vi "test_harness_Sat_op_fxp_16_5.vi"() -> ()   [LabVIEW 2017, in "Sat_Hyst_TestCase.lvclass"]
uses:
  Sat_Hyst_TestCase.lvclass
  C:/Program Files (x86)/National Instruments/LabVIEW 2017/vi.lib/addons/_JKI Toolkits/VI Tester/TestCase.llb/TestCase.lvclass
  <vilib>/rvi/DesktopExecutionNode/Execution/niFpgaDEN_Execute.vi
  <vilib>/rvi/DesktopExecutionNode/DesktopExecutionNode.xnode
  <userlib>/_VITAC/VITAC.lvlib
panel:
  in  "error in (no error)":errorcluster
  out "error out":errorcluster
  out "TestCase out":refnum<class "Sat_Hyst_TestCase.lvclass">
  in  "TestCase in":refnum<class "Sat_Hyst_TestCase.lvclass">
  out "H_of_uk":fxp<+/-,32,10>[](array[numeric])
  out "sat(U) (expected, ML)":dbl[](array[numeric])
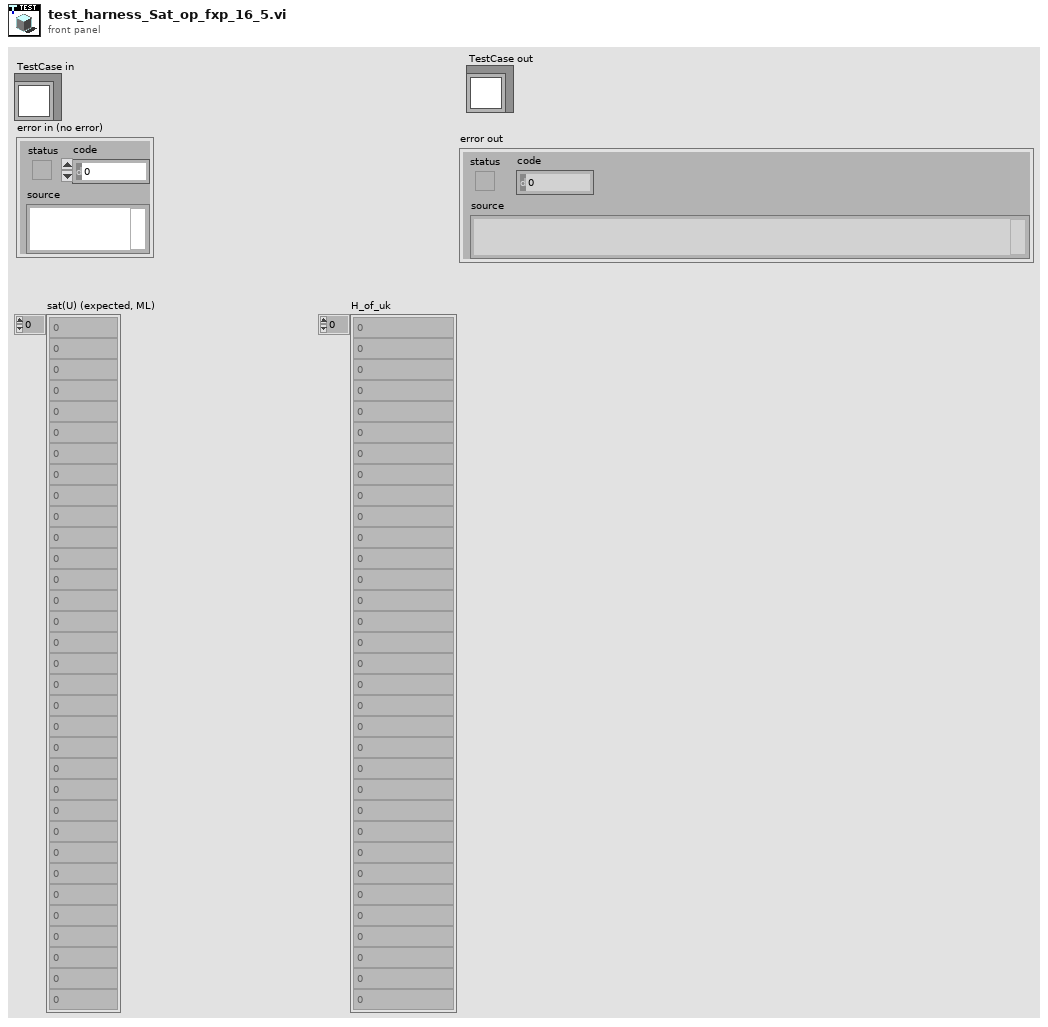
[diagram p1: front panel]
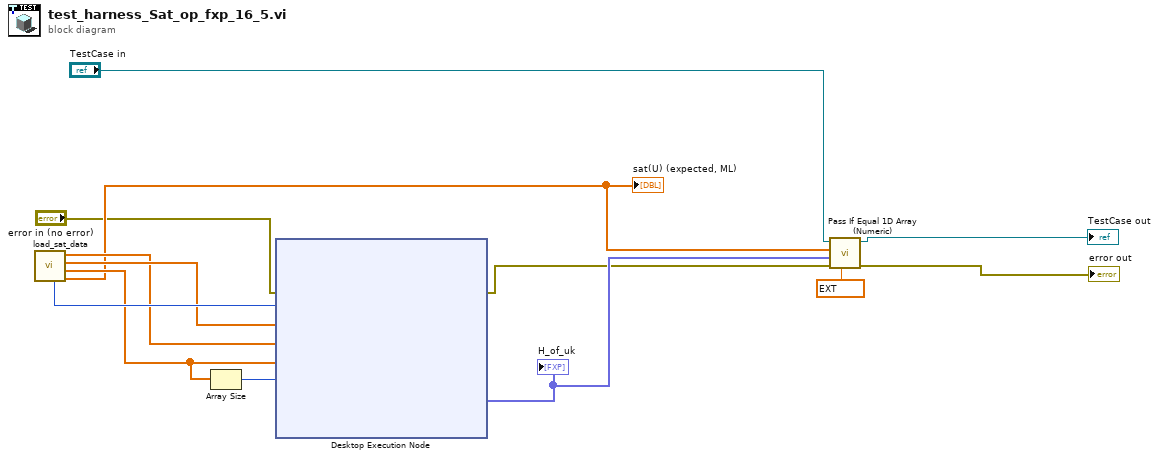
[diagram p0: block diagram]
diagram:
  n1 = call "load_sat_data.vi"() -> ("sat(U_nom)"=w6:dbl[], "U_nom"=w9:dbl[], "wsp"=w12:dbl[], "dps"=w11:dbl[], "N_hyst"=w13:i32)  [unwired: 7 in]
  "sat(U) (expected, ML)" <- w6
  n2 = Array Size(array=w9) -> (size(s)=w10:i32)
  n3 = xnode "Desktop Execution Node"("Error In"="error in (no error)", "N_sat"=w13, "satw_s"=w12, "d_s"=w11, "uk"=w9, "numIter"=w10) -> ("Error Out"=w3:errorcluster, "H_of_uk"=w5:fxp<+/-,32,10>[])  [unwired: 1 out]
  "H_of_uk" <- w5
  n4 = call <userlib>:"Pass If Equal 1D Array (Numeric).vi"("delta (optional)"=ext 0.0001, "error in (no error)"=w3, "actual"=w5, "expected"=w6, "TestCase in"="TestCase in") -> ("error out"=→"error out":errorcluster, "TestCase out"=→"TestCase out":refnum<class "Sat_Hyst_TestCase.lvclass">)  [unwired: 5 in]
